vi "Update Frame Element.vi"(9 "Detection Frame In in":T1 {"robots_blue"."height" format="%+4.3f"; "robots_blue"."pixel_y" format="%+4.3f"; "robots_blue"."pixel_x" format="%+4.3f"; "robots_blue"."orientation" format="%+4.3f"; "robots_blue"."y" format="%+4.3f"; "robots_blue"."confidence" format="%4.3f"; "robots_blue"."x" format="%+4.3f"; "robots_yellow"."height" format="%+4.3f"; "robots_yellow"."pixel_y" format="%+4.3f"; "robots_yellow"."pixel_x" format="%+4.3f"; "robots_yellow"."orientation" format="%+4.3f"; "robots_yellow"."y" format="%+4.3f"; "robots_yellow"."confidence" format="%4.3f"; "robots_yellow"."x" format="%+4.3f"}, 10 "Numeric":i32, 11 "Detection Frame In 3":T1[](array[typedef]) {"robots_blue"."height" format="%+4.3f"; "robots_blue"."pixel_y" format="%+4.3f"; "robots_blue"."pixel_x" format="%+4.3f"; "robots_blue"."orientation" format="%+4.3f"; "robots_blue"."y" format="%+4.3f"; "robots_blue"."confidence" format="%4.3f"; "robots_blue"."x" format="%+4.3f"; "robots_yellow"."height" format="%+4.3f"; "robots_yellow"."pixel_y" format="%+4.3f"; "robots_yellow"."pixel_x" format="%+4.3f"; "robots_yellow"."orientation" format="%+4.3f"; "robots_yellow"."y" format="%+4.3f"; "robots_yellow"."confidence" format="%4.3f"; "robots_yellow"."x" format="%+4.3f"}) -> (3 "Detection Frame In out":T1[](array[typedef]) {"robots_blue"."height" format="%+4.3f"; "robots_blue"."pixel_y" format="%+4.3f"; "robots_blue"."pixel_x" format="%+4.3f"; "robots_blue"."orientation" format="%+4.3f"; "robots_blue"."y" format="%+4.3f"; "robots_blue"."confidence" format="%4.3f"; "robots_blue"."x" format="%+4.3f"; "robots_yellow"."height" format="%+4.3f"; "robots_yellow"."pixel_y" format="%+4.3f"; "robots_yellow"."pixel_x" format="%+4.3f"; "robots_yellow"."orientation" format="%+4.3f"; "robots_yellow"."y" format="%+4.3f"; "robots_yellow"."confidence" format="%4.3f"; "robots_yellow"."x" format="%+4.3f"})   [LabVIEW 2016]
uses:
  SSL Detection Frame.ctl
  SSL Detection Robot.ctl
  <vilib>/Analysis/Matrix/Datatypes/RealMatrix.ctl
  SSL Detection Ball.ctl
  <vilib>/Analysis/Matrix/NI_Matrix.lvlib
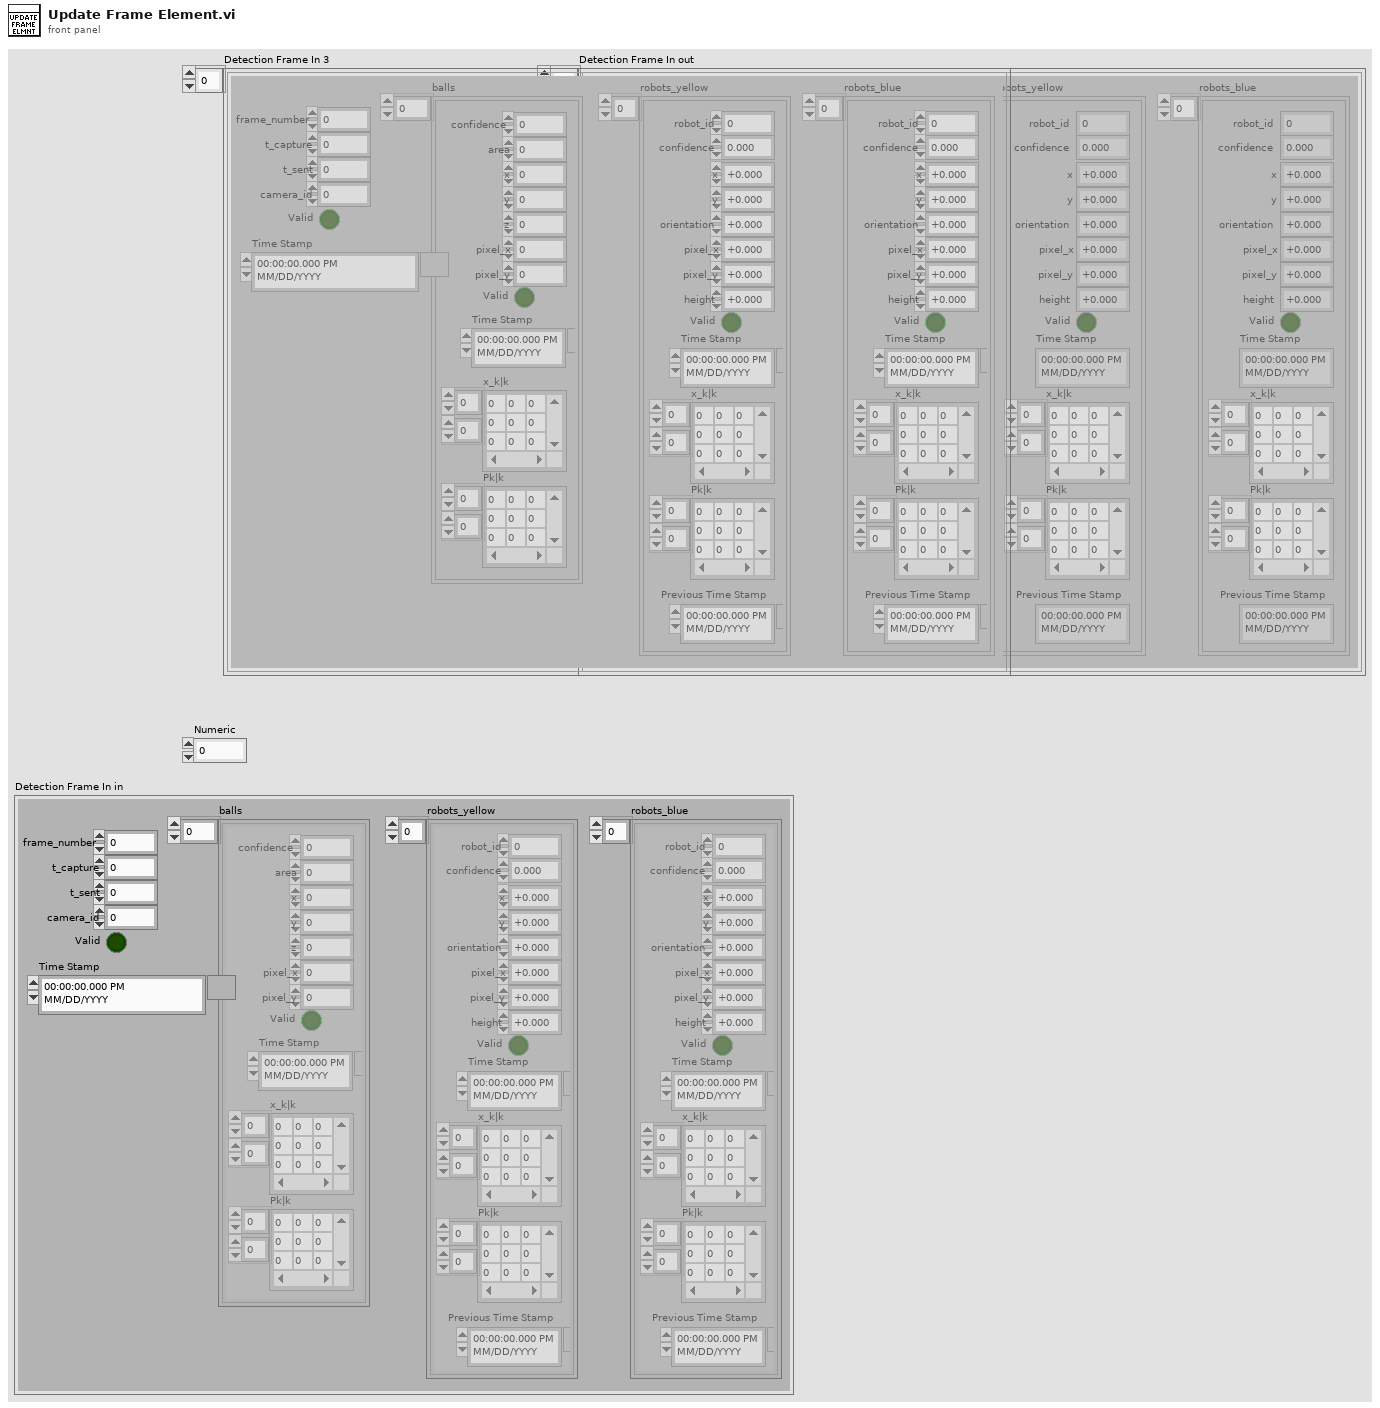
[diagram p1: front panel]
types:
  T1 = typedef "SSL Detection Frame.ctl" = cluster{"frame_number":u32, "t_capture":dbl, "t_sent":dbl, "camera_id":u32, "robots_yellow":T2[], "robots_blue":T2[], "balls":T4[], "Valid":bool, "Time Stamp":timestamp}
  T2 = typedef "SSL Detection Robot.ctl" = cluster{"x":sgl, "robot_id":u32, "confidence":sgl, "y":sgl, "orientation":sgl, "pixel_x":sgl, "pixel_y":sgl, "height":sgl, "Valid":bool, "Time Stamp":timestamp, "x_k|k":T3, "Pk|k":T3, "Previous Time Stamp":timestamp}
  T3 = typedef "NI_Matrix.lvlib/RealMatrix.ctl" = dbl[][]
  T4 = typedef "SSL Detection Ball.ctl" = cluster{"x":sgl, "area":u32, "confidence":sgl, "y":sgl, "z":sgl, "pixel_x":sgl, "pixel_y":sgl, "Valid":bool, "Time Stamp":timestamp, "x_k|k":T3, "Pk|k":T3}
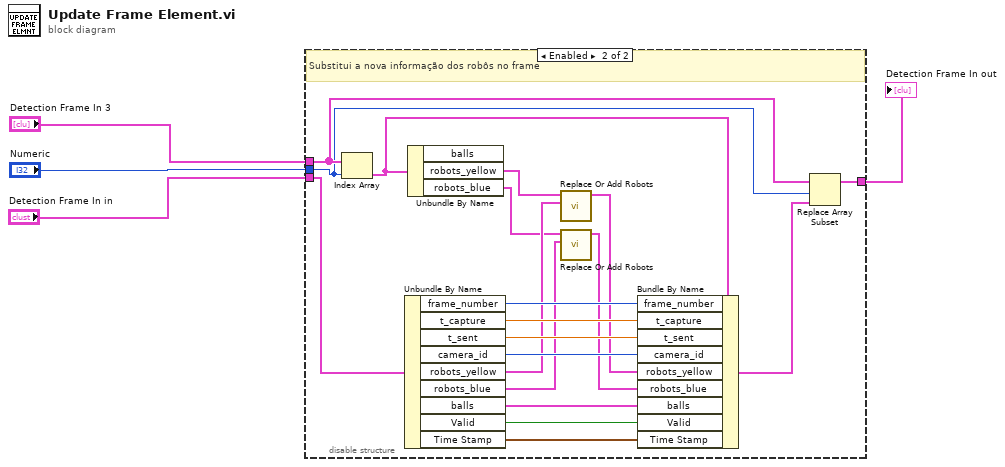
[diagram p0: block diagram]
diagram:
  n1 = disable-structure shown="Enabled" {
    disable-tunnel: "Detection Frame In 3" -> [_ w8]
    disable-tunnel: "Numeric" -> [_ w6]
    disable-tunnel: "Detection Frame In in" -> [_ w22]
    disable-tunnel: [_ w5] -> w4
    frame Disabled {
    }
    frame Enabled {
      # "Substitui a nova informação dos robôs no frame"
      n2 = Index Array(array=w8, index=w6) -> (element=w23:T1)
      n3 = Unbundle By Name(w22) -> ("frame_number"=w21:u32, "t_capture"=w20:dbl, "t_sent"=w19:dbl, "camera_id"=w18:u32, "robots_yellow"=w13:T2[], "robots_blue"=w10:T2[], "balls"=w17:T4[], "Valid"=w16:bool, "Time Stamp"=w15:timestamp)
      n4 = Unbundle By Name(w23) -> ("robots_yellow"=w14:T2[], "robots_blue"=w11:T2[])  [unwired: 1 out]
      n5 = call "Replace Or Add Robots.vi"("Robots New"=w13, "Robots Old"=w14) -> ("Robots New Out"=w12:T2[])  [unwired: 9 in]
      n6 = call "Replace Or Add Robots.vi"("Robots New"=w10, "Robots Old"=w11) -> ("Robots New Out"=w9:T2[])  [unwired: 9 in]
      n7 = Bundle By Name(cluster=w23, "frame_number"=w21, "t_capture"=w20, "t_sent"=w19, "camera_id"=w18, "robots_yellow"=w12, "robots_blue"=w9, "balls"=w17, "Valid"=w16, "Time Stamp"=w15) -> (w7:T1)
      n8 = Replace Array Subset(array=w8, new element=w7, index=w6) -> (w5:T1[])
    }
  }
  "Detection Frame In out" <- w4
